vi "Get System Page Size.vi"(8 "error in (no error)":errorcluster, 11 "shared memory in":T1) -> (0 "error out":errorcluster, 2 "page size (bytes)":u32, 3 "shared memory out":T1)   [LabVIEW 2016, in "Linux RT IPC.Shared Memory.lvlib" / "Shared Memory.lvclass"]
doc: "This VI returns the size of pages in memory for the current system. For most Linux operating systems, this value is 4096 bytes (4kB)."
uses:
  Shared Memory.lvclass
  Controls/reference.ctl
  C/Linux RT IPC.C.lvlib
  Linux RT IPC.Shared Memory.lvlib
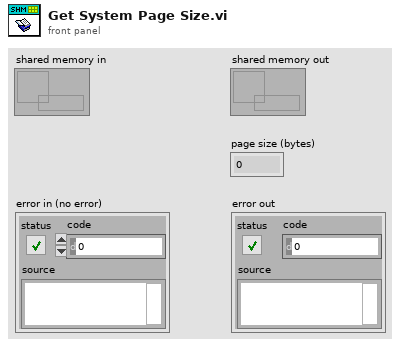
[diagram p1: front panel]
types:
  T1 = typedef "Linux RT IPC.Shared Memory.lvlib/reference.ctl" = refnum<data-value>
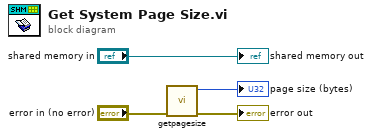
[diagram p0: block diagram]
diagram:
  n1 = call "getpagesize.vi"("error in (no error)"="error in (no error)") -> ("error out"=→"error out":errorcluster, "page size"=→"page size (bytes)":u32)  [unwired: 9 in]
  "shared memory out" <- "shared memory in"
